vi "UE9 Two 32-bit Frequency Measurements.vi"() -> ()   [LabVIEW 2021]
panel:
  in  "Case Constant\n(See Context Help)":bool=TRUE
  in  "DeviceType":u16(ring)=1 items=["LJ_dtU3", "LJ_dtUE9"]
  out "Counter1 Diff (FIO3)":u32
  out "Frequency (FIO1)":dbl format="%.2f"
  out "Period (FIO1)":dbl format="%.6f"
  out "Iteration":i32
  out "Frequency (FIO0)":dbl format="%.2f"
  out "Period (FIO0)":dbl format="%.6f"
  in  "error in":errorcluster
  in  "ConnectionType":u16(ring) items=["LJ_ctUSB", "LJ_ctETHERNET"]
  in  "Address":string="1"
  in  "FirstFound":bool=TRUE
  in  "stop":bool
  out "Counter0 Diff (FIO2)":u32
  out "error out":errorcluster
  out "Error Message":string
  # "Each iteration, this VI measures the frequency on FIO0 and FIO1 using timer mode 2 (32-bit\nperiod measurement).  Also reads the count on FIO2 and FIO3 and\ndisplays the difference from the previous iteration, with the idea that the same signal can\nbe connected to FIO0 and FIO2 (and to FIO1 and FIO3) for comparison of period timing\nversus pulse counting."
  # "seconds"
  # "seconds"
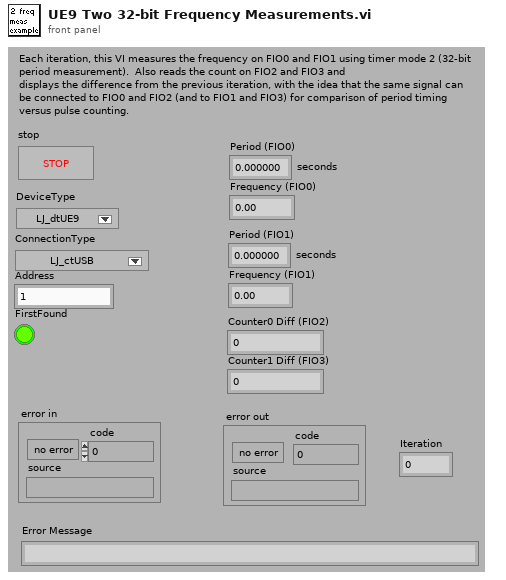
[diagram p1: front panel]
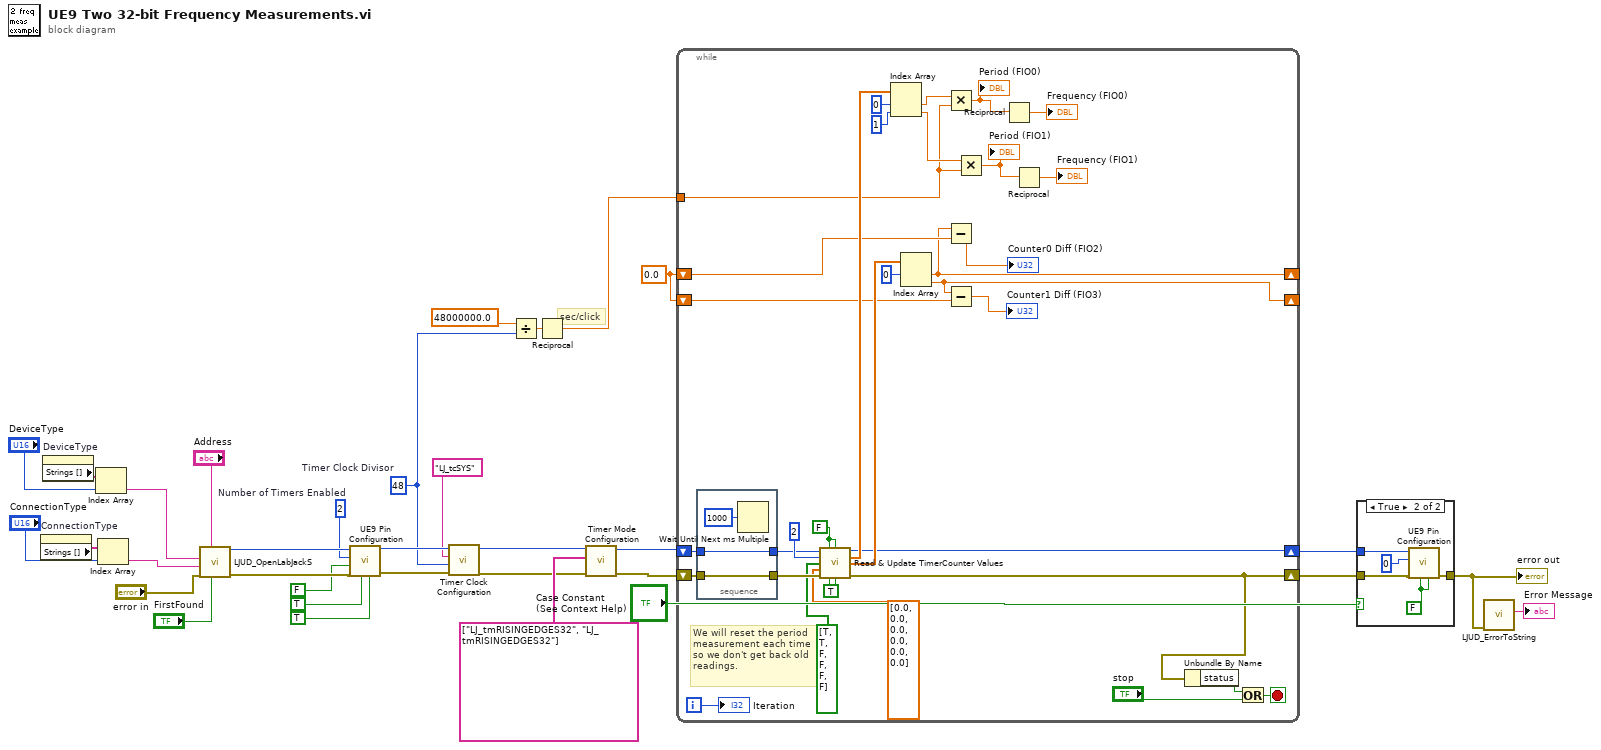
[diagram p0: block diagram]
diagram:
  w1 = 48  # Timer Clock Divisor
  w3 = u8 2  # Number of Timers Enabled
  w22 = 0.0 ("TimerClockConfig")
  # "sec/click"
  n1 = property on="ConnectionType" class="Ring (strict)"() -> ("Strings []"=w20:string[])  [unwired: 2 in, 2 out]
  n2 = property on="DeviceType" class="Ring (strict)"() -> ("Strings []"=w21:string[])  [unwired: 2 in, 2 out]
  n3 = Index Array(array=w21, index="DeviceType") -> (element=w16:string)
  n4 = Index Array(array=w20, index="ConnectionType") -> (element=w17:string)
  n5 = call "LJUD_OpenLabJackS.vi"("FirstFound"="FirstFound", "Address"="Address", "error in"="error in", "ConnectionType"=w17, "DeviceType"=w16) -> ("error out"=w8:errorcluster, "Handle"=w9:i32)  [unwired: 4 in, 1 out]
  n6 = call "UE9 Pin Configuration.vi"("Enable Counter1"=TRUE ("Enable Counter0"), "Enable Counter0"=TRUE, "error in"=w8, "Enable DACs"=FALSE ("Enable Counter0"), "Number of Timers Enabled"=w3, "Handle In"=w9) -> ("error out"=w12:errorcluster, "Handle Out"=w11:i32)  [unwired: 4 in]
  n7 = call "Timer Clock Configuration.vi"("error in"=w12, "Timer Clock Divisor"=w1, "Timer Clock Base"="LJ_tcSYS", "Handle In"=w11) -> ("error out"=w13:errorcluster, "Handle Out"=w10:i32)  [unwired: 6 in]
  n8 = Divide(x=48000000.0, y=w1) -> (x/y=w24:dbl)
  n9 = Reciprocal(x=w24) -> (1/x=w23:dbl)
  n10 = call "Timer Mode Configuration.vi"("error in"=w13, "TimerModes"=string[] ["LJ_tmRISINGEDGES32", "LJ_tmRISINGEDGES32"], "Handle In"=w10) -> ("error out"=w6:errorcluster, "Handle Out"=w7:i32)  [unwired: 7 in]
  n11 = while {
    shift-right: [w36] -> w29
    shift-left: w7 -> [w66]
    shift-right: [w35] -> w30
    shift-left: w6 -> [w65]
    tunnel: w23 -> [w42]
    shift-right: [w48] -> _
    shift-left: w22 -> [w50]
    shift-right: [w38] -> _
    shift-left: w22 -> [w39]
    i -> [w47]
    stop <- w55 stop-if-true
    w34 = TRUE ("Reset Counter0")
    w64 = FALSE ("Reset Counter0")
    # "We will reset the period\nmeasurement each time\nso we don't get back old\nreadings."
    n12 = stacked-sequence {
      tunnel: [w68] -> w60
      tunnel: [w67] -> w59
      tunnel: w66 -> [w68]
      tunnel: w65 -> [w67]
      frame #0 {
        n13 = Wait Until Next ms Multiple(millisecond multiple=u32 1000) -> ()  [unwired: 1 out]
      }
    }
    n14 = call "Read & Update TimerCounter Values.vi"("Handle In"=w60, "Reset Counter0"=w64, "Reset Counter1"=w64, "# Timers to Read"=2, "UpdateReset Timers"=bool[] [TRUE, TRUE, FALSE, FALSE, FALSE, FALSE], "TimerValues"=dbl[] [0.0, 0.0, 0.0, 0.0, 0.0, 0.0], "error in"=w59, "Read Counter0"=w34, "Read Counter1"=w34) -> ("Handle Out"=w36:i32, "Timer Value Reads"=w57:dbl[], "Counter Value Reads"=w62:dbl[], "error out"=w35:errorcluster)  [unwired: 3 in]
    n15 = Index Array(array=w57, index #1=0 ("Index"), index #2=1 ("Index")) -> (element #1=w44:dbl, element #2=w43:dbl)
    n16 = Index Array(array=w62, index #1=0 ("Index")) -> (element #1=w48:dbl, element #2=w38:dbl)  [unwired: 1 in]
    n17 = Multiply(x=w44, y=w42) -> (x*y=w52:dbl)
    "Period (FIO0)" <- w52
    n18 = Subtract(x=w48, y=w50) -> (x-y=→"Counter0 Diff (FIO2)":dbl)
    n19 = Subtract(x=w38, y=w39) -> (x-y=→"Counter1 Diff (FIO3)":dbl)
    n20 = Multiply(x=w43, y=w42) -> (x*y=w46:dbl)
    "Period (FIO1)" <- w46
    n21 = Reciprocal(x=w52) -> (1/x=→"Frequency (FIO0)":dbl)
    n22 = Reciprocal(x=w46) -> (1/x=→"Frequency (FIO1)":dbl)
    n23 = Unbundle By Name(w35) -> ("status"=w54:bool)
    n24 = Or(x=w54, y="stop") -> (x .or. y?=w55:bool)
    "Iteration" <- w47
  }
  n25 = case shown="True" "Case Constant\n(See Context Help)" {
    tunnel: w30 -> [w70 w75]
    tunnel: w29 -> [_ w74]
    tunnel: [w70 w71] -> w32
    frame False {
    }
    frame True {
      w73 = FALSE ("Enable Counter0")
      n26 = call "UE9 Pin Configuration.vi"("Enable Counter1"=w73, "Enable Counter0"=w73, "error in"=w75, "Number of Timers Enabled"=u8 0 ("# Timers Enabled"), "Handle In"=w74) -> ("error out"=w71:errorcluster)  [unwired: 5 in, 1 out]
    }
  }
  "error out" <- w32
  n27 = call "LJUD_ErrorToString.vi"("error in"=w32) -> ("String"=→"Error Message":string)  [unwired: 10 in]
